vi "test5-ChainNodeBroadcast.vi"(8 "error in (no error)":errorcluster, 11 "TestCase in":refnum<class "testcase-CSMChainMode.lvclass">) -> (0 "error out":errorcluster, 3 "TestCase out":refnum<class "testcase-CSMChainMode.lvclass">)   [LabVIEW 2017, in "testcase-CSMChainMode.lvclass"]
uses:
  testcase-CSMChainMode.lvclass
  b9a68168-9423-447a-be7f-8ac0ebad77aa.vi
  a50093c0-808a-49cf-b933-7f76f8d4e341.vi
  src/user.lib/_NEVSTOP/Communicable State Machine(CSM)/AdvanceAPI/CSM - Get Module Attribute.vi
  <vilib>/addons/_JKI Toolkits/VI Tester/TestCase.llb/TestCase.lvclass
  src/user.lib/_NEVSTOP/Communicable State Machine(CSM)/Communicable State Machine.lvlib
  CSM/CSM-Testcase.lvlib
  C:/Program Files (x86)/National Instruments/LabVIEW 2017/vi.lib/addons/_JKI Toolkits/VI Tester/TestCase.llb/TestCase.lvclass
panel:
  out "LoopCount":i32
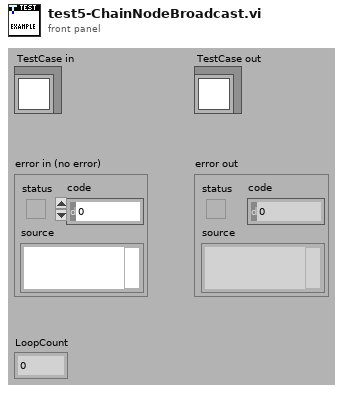
[diagram p1: front panel]
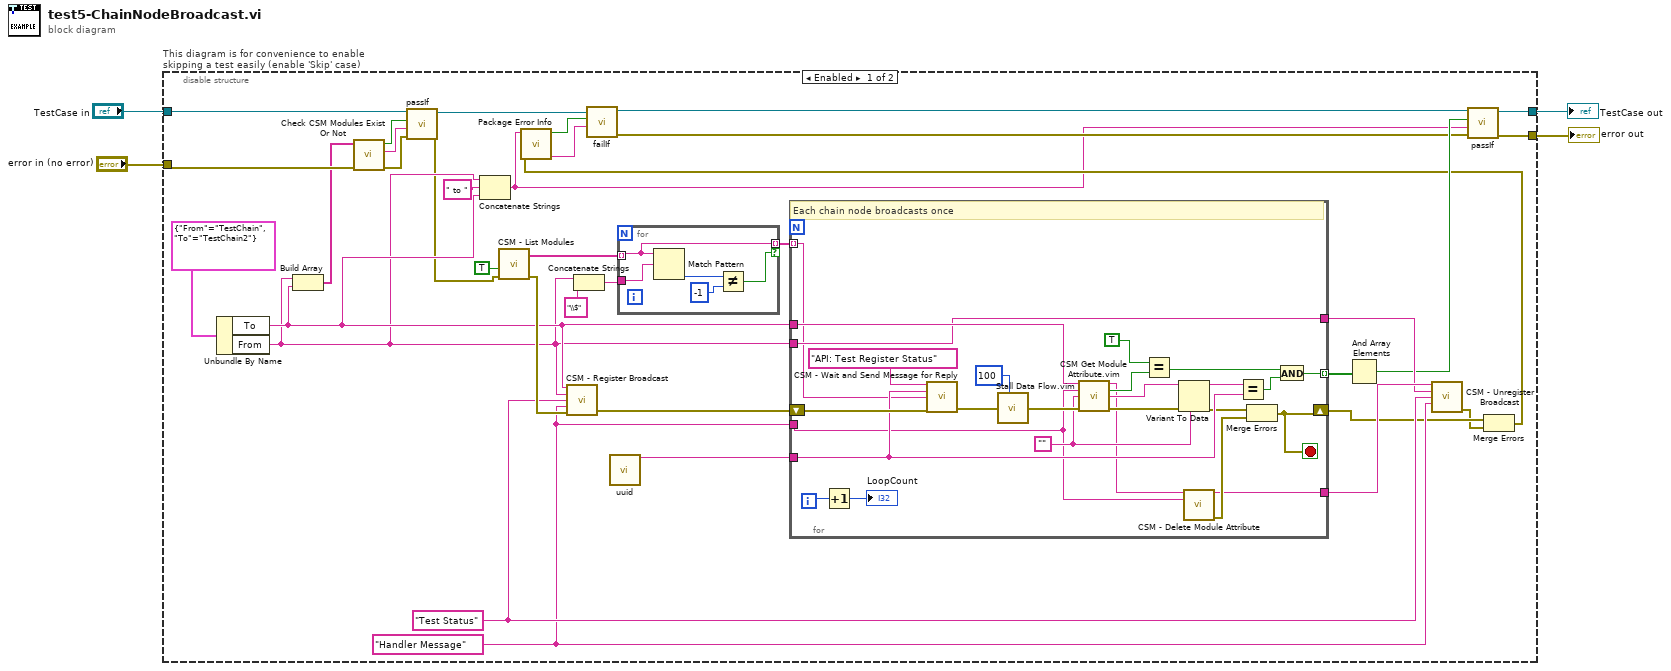
[diagram p0: block diagram]
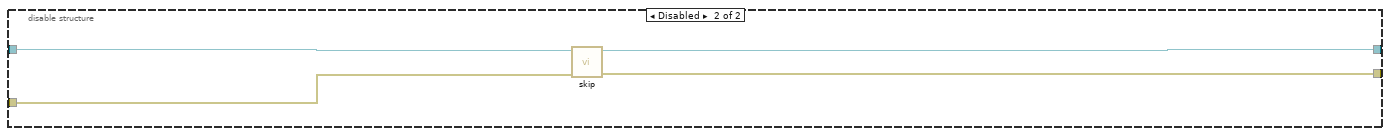
[diagram p2: hidden frame]
diagram:
  n1 = disable-structure "This diagram is for convenience to enable skipping a test easily (enable 'Skip' case)" shown="Enabled" {
    disable-tunnel: "TestCase in" -> [w14 w75]
    disable-tunnel: [w24 w73] -> w1
    disable-tunnel: [w23 w74] -> w3
    disable-tunnel: "error in (no error)" -> [w12 w72]
    frame Enabled {
      w30 = "Handler Message" ("API (If \"\", Same as Trigger)")
      w31 = "Test Status" ("Trigger")
      n2 = Unbundle By Name(cluster{"From":string, "To":string} {"From"="TestChain", "To"="TestChain2"} ("Cluster")) -> ("To"=w10:string, "From"=w9:string)
      n3 = Build Array(w9, w10) -> (w11:string[])
      n4 = call "Check CSM Modules Exist Or Not.vi"("error in"=w12, "CSM names in"=w11) -> ("error out"=w19:errorcluster, "Debug string"=w20:string, "All Modules Exist?"=w21:bool)  [unwired: 7 in]
      n5 = call-dynamic "passIf.vi"("error in (no error)"=w19, "message (\"\")"=w20, "pass"=w21, "TestCase in"=w14) -> ("error out"=w8:errorcluster, "TestCase out"=w15:refnum<class "testcase-CSMChainMode.lvclass">)  [unwired: 6 in]
      n6 = Concatenate Strings(w9, " to " ("string"), w10) -> (w5:string)
      n7 = call "CSM - List Modules.vi"("Error In"=w8, "With Nodes? (F)"=TRUE) -> ("error out"=w33:errorcluster, "Module Names"=w36:string[])  [unwired: 8 in]
      n8 = call "CSM - Register Broadcast.vi"("CSM Name(Empty for Broadcast Event)"=w10, "Source CSM Name (* as Default)"=w9, "Trigger"=w31, "API (If \"\", Same as Trigger)"=w30, "Error In"=w33) -> ("error out"=w35:errorcluster)  [unwired: 9 in, 1 out]
      n9 = Concatenate Strings(w9, "\\$" ("string")) -> (w38:string)
      n10 = call "uuid.vi"() -> ("UUID"=w34:string)  [unwired: 11 in]
      n11 = for {
        tunnel: w36 -> [w69] mode=indexing
        tunnel: [w69] -> w32 mode=indexing if=w68
        tunnel: w38 -> [w67]
        n12 = Match Pattern(string=w69, regular expression=w67) -> (offset past match=w71:i32)  [unwired: 1 in, 3 out]
        n13 = Not Equal?(x=w71, y=-1) -> (x != y?=w68:bool)
      }
      n14 = for {
        tunnel: w34 -> [w52]
        tunnel: w32 -> [w42] mode=indexing
        tunnel: w10 -> [w59]
        tunnel: w30 -> [w48]
        shift-right: [w41] -> w27
        shift-left: w35 -> [w65]
        tunnel: w9 -> [w43]
        tunnel: [w45] -> w29
        tunnel: [w43] -> w28
        tunnel: [w44] -> w25 mode=indexing
        i -> [w64]
        stop <- w41 stop-if-true
        w54 = ""
        # "Each chain node broadcasts once"
        n15 = Increment(x=w64) -> (x+1=→"LoopCount":i32)
        n16 = call "CSM - Wait and Send Message for Reply.vi"("State"="API: Test Register Status", "Arguments (\"\")"=w52, "Target Module"=w42, "Error In (No Error)"=w65) -> ("error out"=w62:errorcluster)  [unwired: 8 in, 3 out]
        n17 = call "Stall Data Flow.vim"("value in"=w62, "milliseconds to wait"=u32 100) -> ("value out"=w60:errorcluster)  [unwired: 1 out]
        n18 = call "CSM Get Module Attribute.vim"("CSM Name"=w59, "Attribute"=w48, "Default Value (Empty Variant)"=w54, "Error In"=w60) -> ("CSM Name (Dup)"=w49:string, "Found"=w57:bool, "Value"=w55:string, "error out"=w56:errorcluster)  [unwired: 7 in, 1 out]
        n19 = Equal?(x=TRUE, y=w57) -> (x = y?=w50:bool)
        n20 = Variant To Data(error in=w56, type=w54, Variant=w55) -> (data=w53:string, error out=w47:errorcluster)
        n21 = call "CSM - Delete Module Attribute.vi"("CSM Name"=w49, "Attribute"=w48) -> ("CSM Name (Dup)"=w45:string, "error out"=w46:errorcluster)  [unwired: 10 in, 2 out]
        n22 = Equal?(x=w53, y=w52) -> (x = y?=w51:bool)
        n23 = Merge Errors(w47, w46) -> (w41:errorcluster)
        n24 = And(x=w50, y=w51) -> (x .and. y?=w44:bool)
      }
      n25 = And Array Elements(Boolean array=w25) -> (logical AND=w22:bool)
      n26 = call "CSM - Unregister Broadcast.vi"("CSM Name(Empty for Broadcast Event)"=w29, "Source CSM Name (* as Default)"=w28, "Trigger"=w31, "API (\"*\" as Default)"=w30) -> ("error out"=w26:errorcluster)  [unwired: 10 in, 1 out]
      n27 = Merge Errors(w27, w26) -> (w7:errorcluster)
      n28 = call "Package Error Info.vi"("error in"=w7, "String in"=w5) -> ("packed error info out"=w17:string, "error status"=w18:bool)  [unwired: 8 in]
      n29 = call-dynamic "failIf.vi"("message (\"\")"=w17, "fail"=w18, "TestCase in"=w15) -> ("error out"=w6:errorcluster, "TestCase out"=w13:refnum<class "testcase-CSMChainMode.lvclass">)  [unwired: 7 in]
      n30 = call-dynamic "passIf.vi"("error in (no error)"=w6, "message (\"\")"=w5, "pass"=w22, "TestCase in"=w13) -> ("error out"=w23:errorcluster, "TestCase out"=w24:refnum<class "testcase-CSMChainMode.lvclass">)  [unwired: 6 in]
    }
    frame Disabled {
      # "skip test result while test is under development"
      n31 = call <vilib>:"skip.vi"("error in (no error)"=w72, "TestCase in"=w75) -> ("error out"=w74:errorcluster, "TestCase out"=w73:refnum<class "testcase-CSMChainMode.lvclass">)  [unwired: 8 in]
    }
  }
  "error out" <- w3
  "TestCase out" <- w1
